vi "Write bool_setting.vi"(10 "bool_setting":T1, 11 "Sig_DA in":refnum<class "DA.lvclass">) -> (3 "Sig_DA out":refnum<class "DA.lvclass">)   [LabVIEW 2019]
uses:
  DA.lvclass
  C:/Users/H4001/Documents/GitHub/H4000/src/Signal_class/Signal.lvclass
  C:/Users/H4001/Documents/GitHub/H4000/src/Proccess_class/Proccess.lvclass
  TypeDef/bool_setting.ctl
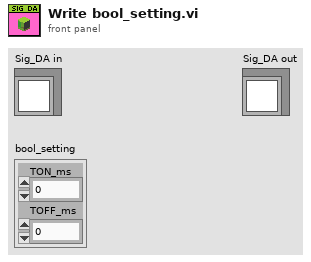
[diagram p1: front panel]
types:
  T1 = typedef "bool_setting.ctl" = cluster{"TON_ms":u32, "TOFF_ms":u32}
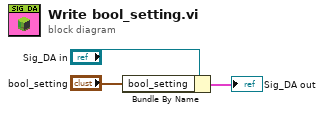
[diagram p0: block diagram]
diagram:
  n1 = Bundle By Name(cluster="Sig_DA in", "bool_setting"="bool_setting") -> (→"Sig_DA out":cluster{})
